vi "getXMLReverse.vi"(8 "error in":errorcluster, 11 "Node":refnum<k20>) -> (0 "error out":errorcluster, 3 "Reverse":cluster{"Reverse X":bool, "Reverse Y":bool})   [LabVIEW 2013]
uses:
  <vilib>/xml/NI_XML.lvlib
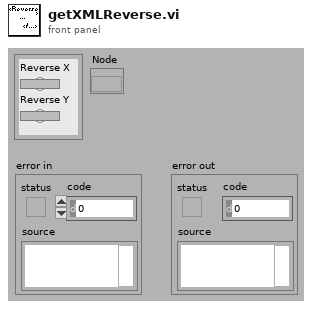
[diagram p1: front panel]
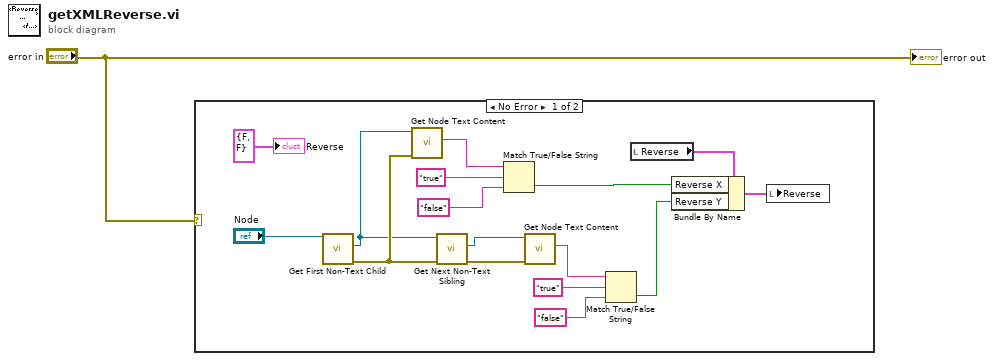
[diagram p0: block diagram]
diagram:
  n1 = case shown="No Error" "error in" {
    frame No Error {
      n2 = call <vilib>:"Get First Non-Text Child.vi"("node in"="Node") -> ("error out"=w5:errorcluster, "child node"=w2:refnum<k20>)  [unwired: 7 in, 2 out]
      n3 = call <vilib>:"Get Node Text Content.vi"("error in (no error)"=w5, "node in"=w2) -> ("node text"=w17:string)  [unwired: 7 in, 2 out]
      n4 = call <vilib>:"Get Next Non-Text Sibling.vi"("error in (no error)"=w5, "node in"=w2) -> ("error out"=w4:errorcluster, "sibling node"=w3:refnum<k20>)  [unwired: 6 in, 2 out]
      n5 = Match True/False String(2:"false" ("false string"), 3:"true" ("true string"), 4:w17) -> (0:w9:bool)  [unwired: 1 out]
      n6 = call <vilib>:"Get Node Text Content.vi"("error in (no error)"=w4, "node in"=w3) -> ("node text"=w12:string)  [unwired: 7 in, 2 out]
      n7 = Match True/False String(2:"false" ("false string"), 3:"true" ("true string"), 4:w12) -> (0:w8:bool)  [unwired: 1 out]
      n8 = local read "Reverse"() -> (w10:cluster{"Reverse X":bool, "Reverse Y":bool})
      n9 = Bundle By Name(cluster=w10, "Reverse X"=w9, "Reverse Y"=w8) -> (w7:cluster{"Reverse X":bool, "Reverse Y":bool})
      n10 = local write "Reverse"(w7) -> ()
      "Reverse" <- cluster{"Reverse X":bool, "Reverse Y":bool} {"Reverse X"=FALSE, "Reverse Y"=FALSE} ("Reverse")
    }
    frame Error {
    }
  }
  "error out" <- "error in"
